vi "fgv.vi"(8 "error in (no error)":errorcluster, 11 "action":T1=enum."get") -> (0 "error out":errorcluster, 3 "dvr":refnum<data-value>)   [LabVIEW 2024, in "controls manager.lvlib"]
uses:
  controls manager.lvlib
  fgv actions.ctl
  collection type.ctl
  entry type.ctl
  control.ctl
  controls plan.ctl
  key value pair.ctl
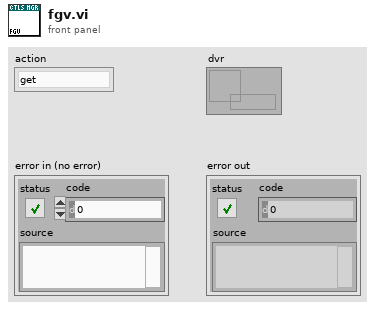
[diagram p1: front panel]
types:
  T1 = typedef "controls manager.lvlib/fgv actions.ctl" = enum16{"create", "get", "destroy"}
  T2 = typedef "controls manager.lvlib/collection type.ctl" = map{string, T3}
  T3 = typedef "controls manager.lvlib/entry type.ctl" = cluster{"controls":map{string, T4}, "plan":T5}
  T4 = typedef "controls manager.lvlib/control.ctl" = cluster{"refnum":refnum<vi>, "index":i32}
  T5 = typedef "controls manager.lvlib/controls plan.ctl" = map{string, T6[]}
  T6 = typedef "controls manager.lvlib/key value pair.ctl" = cluster{"key":string, "value":string}
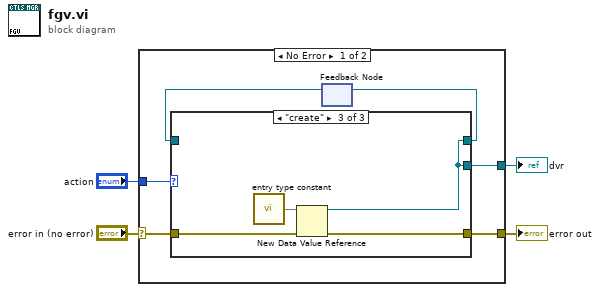
[diagram p0: block diagram]
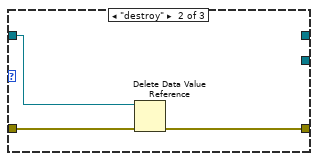
[diagram p3: hidden frame]
diagram:
  n1 = case shown="No Error" "error in (no error)" {
    selector: "error in (no error)" -> [w7 w20]
    tunnel: [w5 _] -> w1
    tunnel: "action" -> [w8 _]
    tunnel: [w6 w20] -> w2
    frame No Error {
      n2 = feedback #1() -> (w9:refnum<data-value>)  [unwired: 1 in]
      n3 = case shown="\"create\"" w8 {
        tunnel: [w12 _ w19] -> w10
        tunnel: w9 -> [w12 w15 _]
        tunnel: [w12 _ w19] -> w5
        tunnel: w7 -> [w11 w14 w18]
        tunnel: [w11 w13 w17] -> w6
        frame "get" {
        }
        frame "destroy" {
          n4 = Delete Data Value Reference(data value reference=w15, error in=w14) -> (error out=w13:errorcluster)  [unwired: 1 out]
        }
        frame "create" {
          n5 = call "entry type constant.vi"() -> ("map"=w16:T2)
          n6 = New Data Value Reference(data value=w16, error in=w18) -> (data value reference=w19:refnum<data-value>, error out=w17:errorcluster)
        }
      }
      n7 = feedback-in #1(w10) -> ()
    }
    frame Error {
    }
  }
  "error out" <- w2
  "dvr" <- w1
